vi "Waveform - Normalize.vi"() -> ()   [LabVIEW 2023]
doc: "Shows how to normalize a waveform to +/- 1."
panel:
  out "Normalized Waveform":waveform(dbl)(graph)
  out "Initial Waveform":waveform(dbl)(graph)
  out "Offset":dbl
  out "Scale":dbl
  # "Overview: Demonstrates how to use the Normalize Waveform VI to modify a waveform so that its maximum value is '1' and its minimum value is '-1'.\nInstructions:\nRun the VI. A Normalized Waveform will be generated. The Scale value indicates the factor by which the waveform was multiplied, and the Offset value indicates the amount the waveform was shifted."
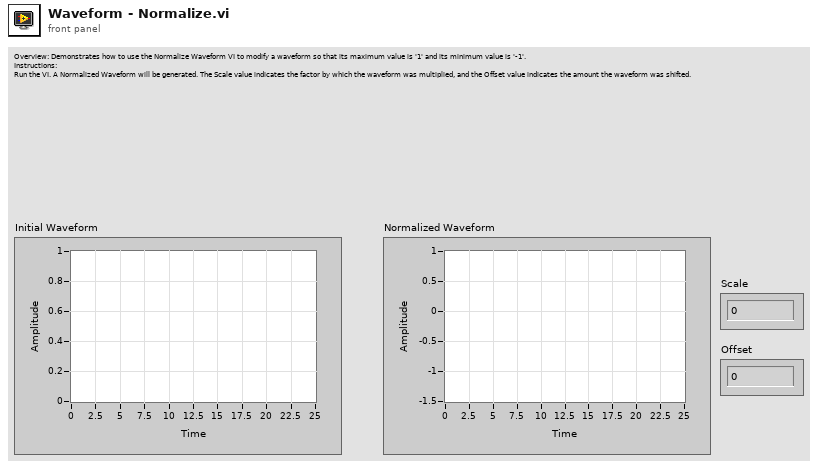
[diagram p1: front panel]
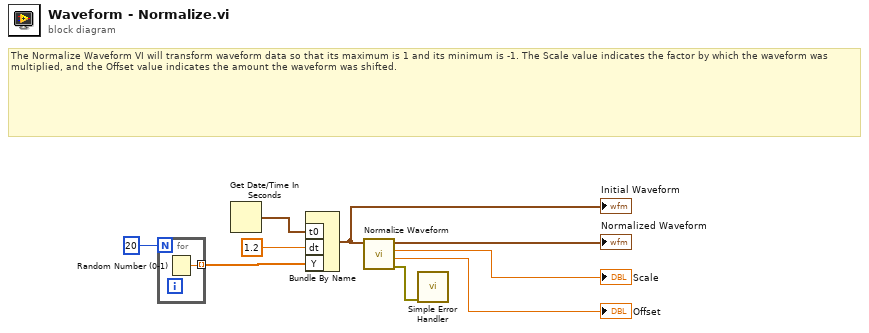
[diagram p0: block diagram]
diagram:
  # "The Normalize Waveform VI will transform waveform data so that its maximum is 1 and its minimum is -1. The Scale value indicates the factor by which the waveform was multiplied, and the Offset value indicates the amount the waveform was shifted."
  n1 = for {
    N: 20 -> [_]
    tunnel: [w10] -> w7 mode=indexing
    n2 = Random Number (0-1)() -> (number: 0 to 1=w10:dbl)
  }
  n3 = Get Date/Time In Seconds() -> (seconds since 1Jan1904=w2:timestamp)
  n4 = Bundle By Name("t0"=w2, "dt"=1.2, "Y"=w7) -> (w4:waveform(dbl))  [unwired: 1 in]
  "Initial Waveform" <- w4
  n5 = call <vilib>:"Normalize Waveform.vi"("waveform in"=w4) -> ("error out"=w1:errorcluster, "offset"=→"Offset":dbl, "scale"=→"Scale":dbl, "normalized waveform"=→"Normalized Waveform":waveform(dbl))  [unwired: 7 in]
  n6 = call <vilib>:"Simple Error Handler.vi"("error in (no error)"=w1) -> ()  [unwired: 4 in, 5 out]
